vi "thermo_reopen.vi"(8 "error in":errorcluster, 10 "allow reopen":bool, 11 "thermo in":T1={"type"=enum."COMET Tx5xx (ethernet)", "comment"="", "tag"="", "refresh"=5.0, "IP"="192.168.2.34", "port"=502, "VISA"="", "last readout"=timestamp(0 s since 1904-01-01), "TCP ref"=refnum, "VISA sess"="", "idn"="", "press"=0.0, "RH"=0.0, "temp"=0.0, "pres cor"=[], "RH cor"=[], "temp cor"=[], "try left"=0, "failed"=FALSE, "RTD set"=[], "RTD inv"=[], "range"=0.0, "net mode"=enum."MODBUS", "try fail"=enum."Stop trying - return NaN", "timeout [s]"=0.0, "max retries"=0, "sim t [deg]"=0.0, "status"=0} {"status" items=["ok", "retry", "failed"]; "RTD inv" format="%.1f"; "RTD set" format="%.1f"; "temp cor" format="%.1f"; "RH cor" format="%.1f"; "pres cor" format="%.1f"; "refresh" min=0.1 max=1000.0 format="%.2f"}) -> (0 "error out":errorcluster, 2 "reopen ok":bool, 3 "thermo out":T1={"type"=enum."COMET Tx5xx (ethernet)", "comment"="", "tag"="", "refresh"=5.0, "IP"="192.168.2.34", "port"=502, "VISA"="", "last readout"=timestamp(0 s since 1904-01-01), "TCP ref"=refnum, "VISA sess"="", "idn"="", "press"=0.0, "RH"=0.0, "temp"=0.0, "pres cor"=[], "RH cor"=[], "temp cor"=[], "try left"=0, "failed"=FALSE, "RTD set"=[], "RTD inv"=[], "range"=0.0, "net mode"=enum."MODBUS", "try fail"=enum."Stop trying - return NaN", "timeout [s]"=0.0, "max retries"=0, "sim t [deg]"=0.0, "status"=0} {"status" items=["ok", "retry", "failed"]; "RTD inv" format="%.1f"; "RTD set" format="%.1f"; "temp cor" format="%.1f"; "RH cor" format="%.1f"; "pres cor" format="%.1f"; "refresh" min=0.1 max=1000.0 format="%.2f"})   [LabVIEW 2020]
uses:
  thermo.ctl
  thermo_types.ctl
  Thermometer Fail Action.ctl
panel:
  out "reopen error out":errorcluster
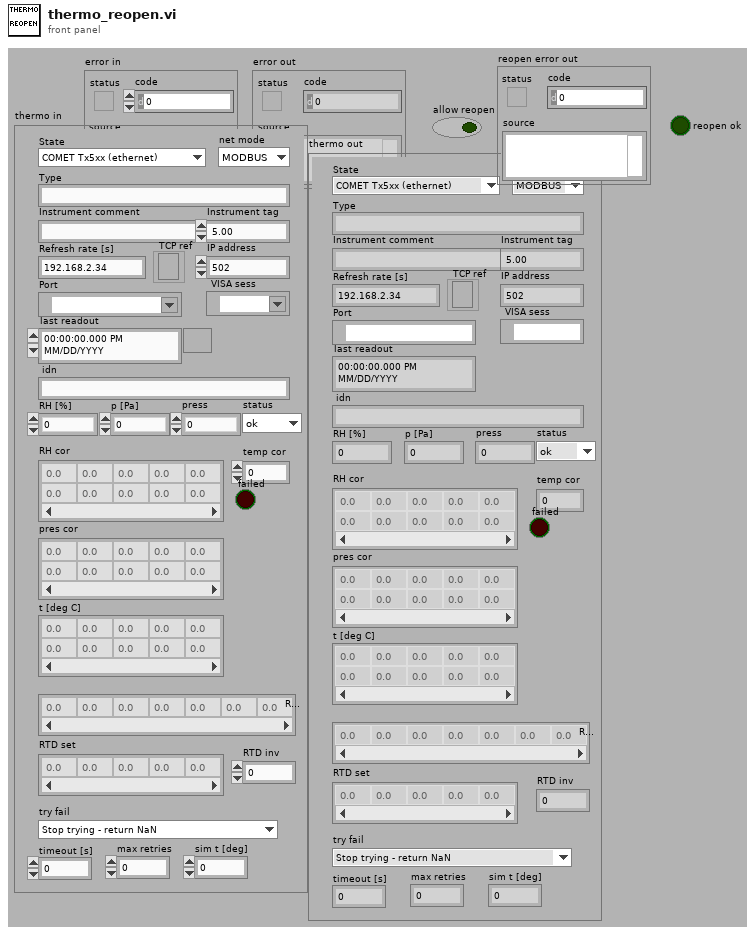
[diagram p1: front panel]
types:
  T1 = typedef "thermo.ctl" = cluster{"type":T2, "comment":string, "tag":string, "refresh":dbl, "IP":string, "port":u16, "VISA":refnum<visa-resource-name>, "last readout":timestamp, "TCP ref":refnum<k5>, "VISA sess":refnum<visa-resource-name>, "idn":string, "press":dbl, "RH":dbl, "temp":dbl, "pres cor":dbl[][], "RH cor":dbl[][], "temp cor":dbl[][], "try left":i32, "failed":bool, "RTD set":dbl[], "RTD inv":dbl[], "range":dbl, "net mode":enum16{"MODBUS", "HTTP"}, "try fail":T3, "timeout [s]":dbl, "max retries":i32, "sim t [deg]":dbl, "status":u16}
  T2 = typedef "thermo_types.ctl" = enum16{"Disabled", "Simulated", "COMET Tx5xx (ethernet)", "Keithley 2002 (GPIB) + RTD", "Agilent 344xx (GPIB) + RTD"}
  T3 = typedef "Thermometer Fail Action.ctl" = enum16{"Stop trying - keep last value", "Stop trying - return NaN", "Generate error - stop sweep"}
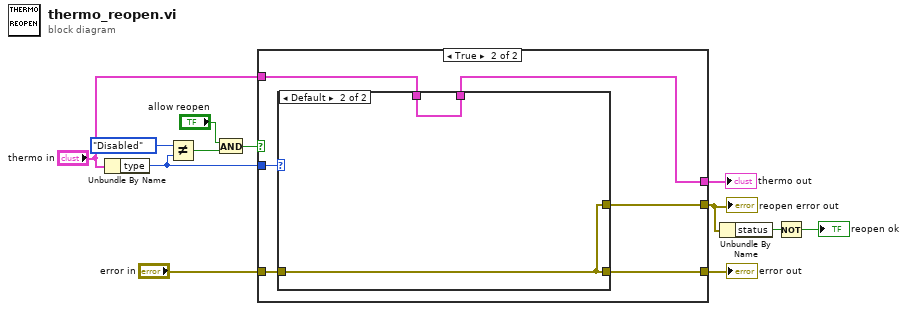
[diagram p0: block diagram]
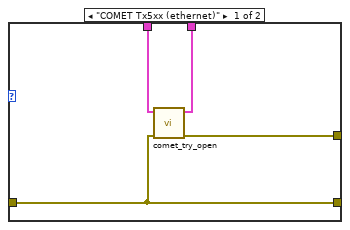
[diagram p3: hidden frame]
diagram:
  n1 = Unbundle By Name("thermo in") -> ("type"=w3:T2)
  n2 = Not Equal?(x=thermo_types."Disabled", y=w3) -> (x != y?=w2:bool)
  n3 = And(x="allow reopen", y=w2) -> (x .and. y?=w8:bool)
  n4 = case shown="True" w8 {
    tunnel: [w13 w18] -> w11
    tunnel: "error in" -> [w13 w19]
    tunnel: w3 -> [_ w20]
    tunnel: "thermo in" -> [w14 w16]
    tunnel: [w14 w15] -> w9
    tunnel: [w13 w17] -> w6
    frame False {
    }
    frame True {
      n5 = case shown="Default" w20 {
        tunnel: [w23 w26] -> w18
        tunnel: w19 -> [w23 w26]
        tunnel: [w24 w26] -> w17
        tunnel: w16 -> [w22 w25]
        tunnel: [w21 w25] -> w15
        frame "COMET Tx5xx (ethernet)" {
          n6 = call "comet_try_open.vi"("error in"=w23, "thermo in"=w22) -> ("error out"=w24:errorcluster, "thermo cluster"=w21:T1)  [unwired: 7 in, 1 out]
        }
        frame Default {
        }
      }
    }
  }
  "error out" <- w11
  "thermo out" <- w9
  "reopen error out" <- w6
  n7 = Unbundle By Name(w6) -> ("status"=w5:bool)
  n8 = Not(x=w5) -> (.not. x?=→"reopen ok":bool)
